vi "FIFO Flush-core.vi"(8 "Error In":errorcluster, 11 "FPGA VI Ref":T1) -> (0 "Error Out":errorcluster, 2 "Ch0 Elements Remaining":u32, 3 "FPGA VI Reference Out":T1)   [LabVIEW 2017]
uses:
  RIG-SPECIFIC FILES/FPGA Refs/FPGA Ref.ctl
  <vilib>/Utility/error.llb/Error Cluster From Error Code.vi
  <vilib>/rvi/errors/niLvFpgaAdjustHostInterfaceError.vi
  <vilib>/rvi/interface/nirviReadWriteControl/nirviReadWriteControl.xnode
  <vilib>/rvi/interface/nirviMethod/nirviMethod.xnode
  <vilib>/rvi/errors/niLvFpgaMergeErrorWithErrorCode.vi
  <vilib>/FPGAPlugInAG/Dynamic/niLvFpga_ReadFifo_Dynamic.vi
  NiFpgaLv.dll
  <vilib>/rvi/interface/Simulation/niFpgaSimulationCallBeginRW.vi
panel:
  out "Loop time array size":i32
  out "Ch1 cleared elements":u32[](array[numeric])
  out "Ch0 Cleared elements":u32[](array[numeric])
  out "Flush Completed":bool
  out "x pixels count":u16[](array[numeric])
  out "y count array":u16[](array[numeric])
  out "x pixels current":u16
  out "y count":u16
  out "Loop Time Array":u32[](array[numeric])
  out "Image time zero":u32
  out "Data Image Time":u64[](array[numeric])
  out "Data Ref Time FIFO":u64[](array[numeric])
  out "Ref time zero":u32
  out "Data Ch1":u32[](array[numeric])
  out "Ch1 Elements Remaining":u32
  out "Data Ch0":u32[](array[numeric])
  in  "Manual force stop":bool
  out "Loop":i32
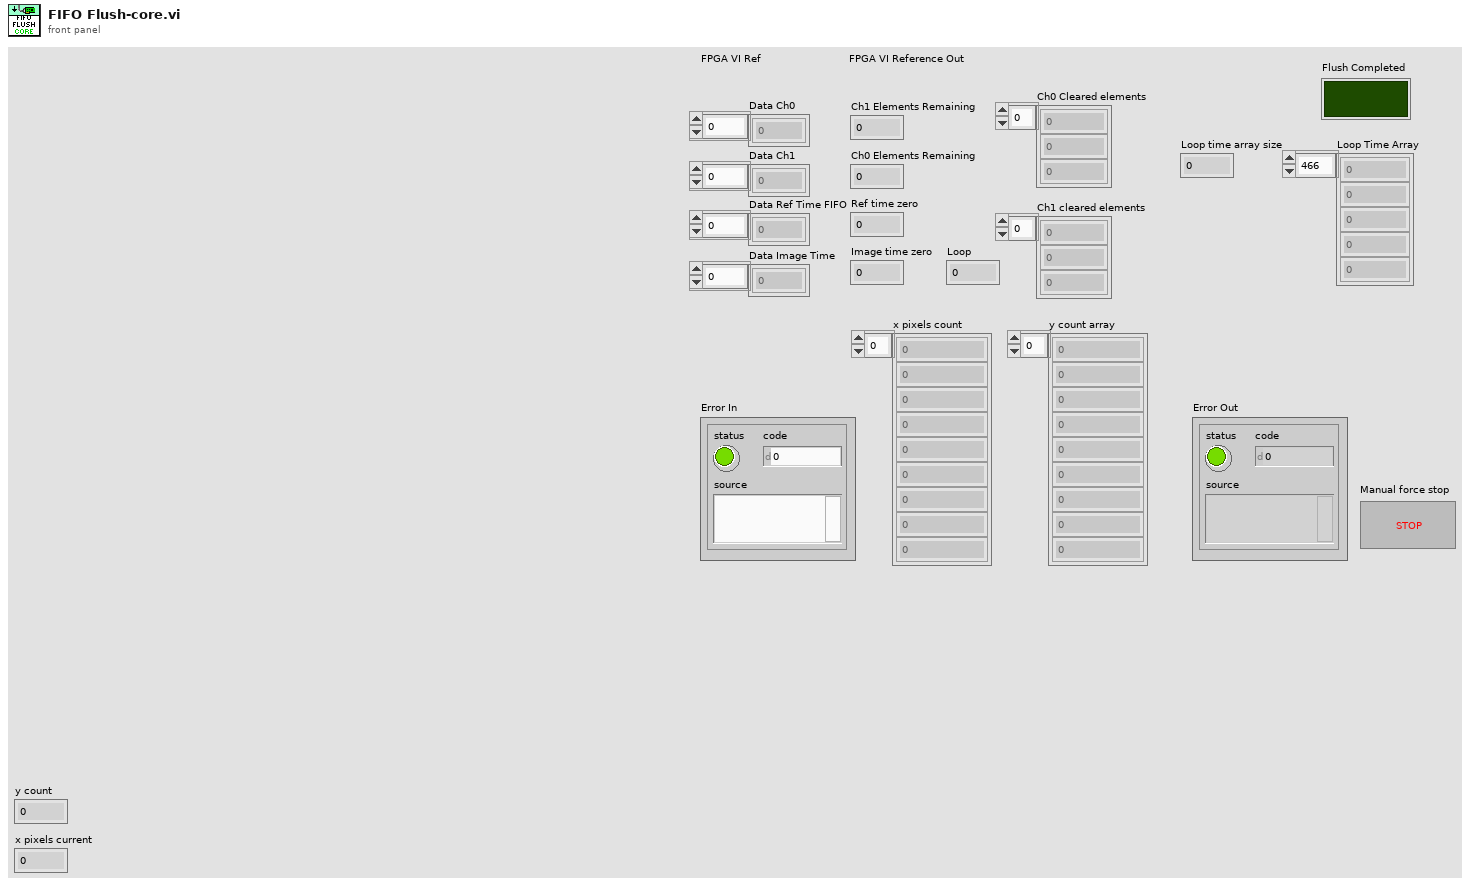
[diagram p1: front panel]
types:
  T1 = typedef "FPGA Ref.ctl" = refnum<k20>
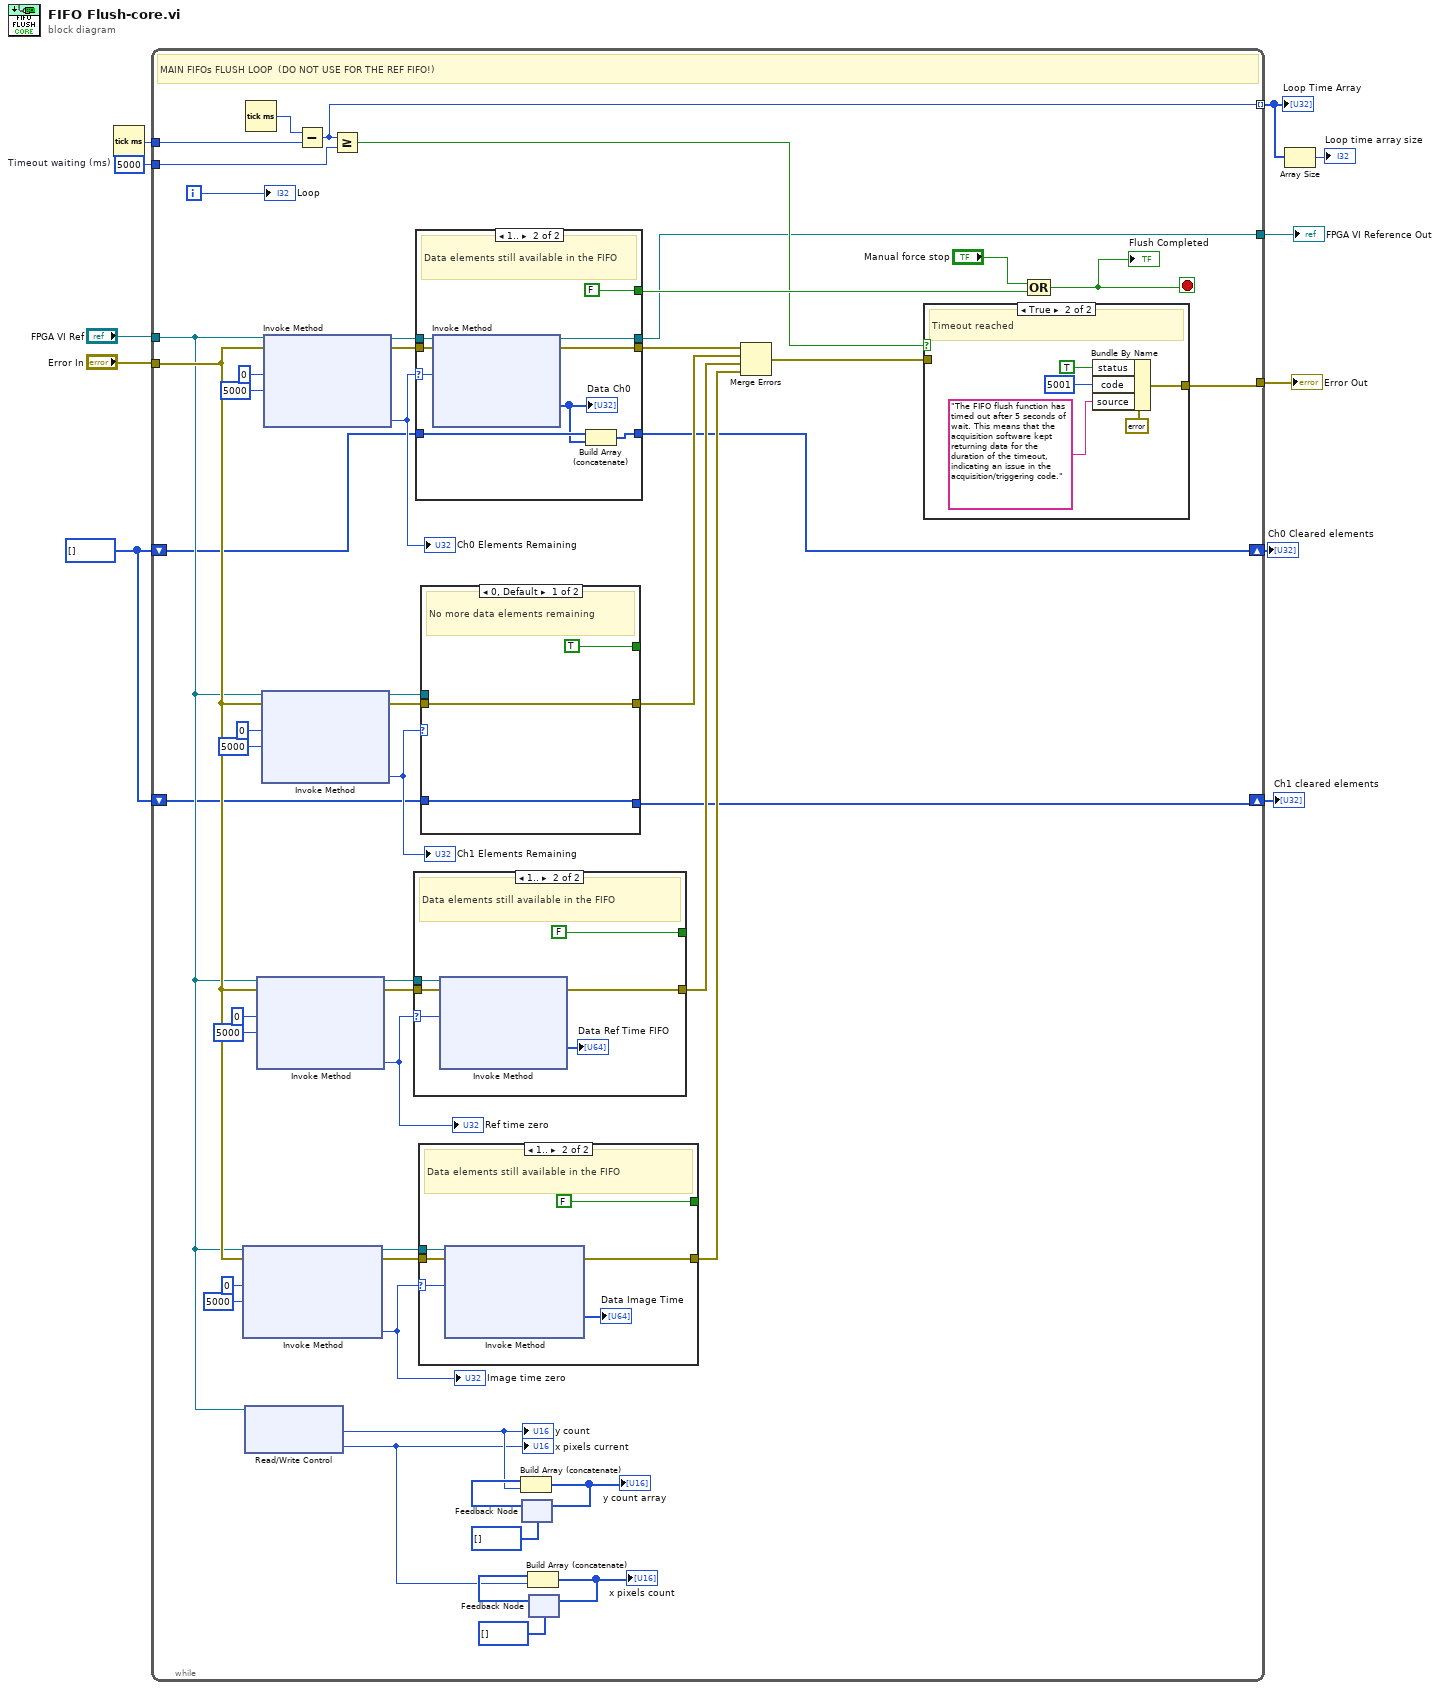
[diagram p0: block diagram]
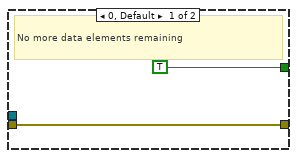
[diagram p2: hidden frame]
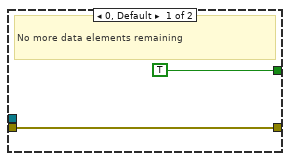
[diagram p3: hidden frame]
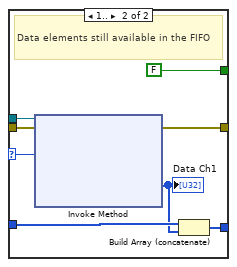
[diagram p4: hidden frame]
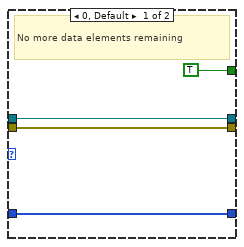
[diagram p6: hidden frame]
diagram:
  w4 = u32[] []
  w7 = u32 5000  # Timeout waiting (ms)
  n1 = Tick Count (ms)() -> (millisecond timer value=w6:u32)
  n2 = while {
    tunnel: "Error In" -> [w27]
    tunnel: [w54] -> w10
    tunnel: w6 -> [w57]
    tunnel: w7 -> [w55]
    tunnel: "FPGA VI Ref" -> [w17]
    tunnel: [w40] -> w8
    tunnel: [w26] -> w2 mode=indexing
    shift-right: [w14] -> w5
    shift-left: w4 -> [w15]
    shift-right: [w12] -> w3
    shift-left: w4 -> [w13]
    i -> [w61]
    stop <- w16 stop-if-true
    # "MAIN FIFOs FLUSH LOOP  (DO NOT USE FOR THE REF FIFO!)"
    n3 = xnode "Invoke Method"("FPGA VI Reference In"=w17, "error in"=w27, "Number of Elements"=u32 0, "Timeout (ms)"=5000) -> ("FPGA VI Reference Out"=w33:T1, "error out"=w34:errorcluster, "Elements Remaining"=w30:u32)  [unwired: 1 out]
    "Image time zero" <- w30
    n4 = xnode "Read/Write Control"("FPGA VI Reference In"=w17) -> ("y count"=w23:u16, "x pixels current"=w18:u16)  [unwired: 1 in, 2 out]
    "y count" <- w23
    "x pixels current" <- w18
    n5 = Tick Count (ms)() -> (millisecond timer value=w58:u32)
    n6 = xnode "Invoke Method"("FPGA VI Reference In"=w17, "error in"=w27, "Number of Elements"=u32 0, "Timeout (ms)"=5000) -> ("FPGA VI Reference Out"=w36:T1, "error out"=w35:errorcluster, "Elements Remaining"=w39:u32)  [unwired: 1 out]
    "Ref time zero" <- w39
    n7 = xnode "Invoke Method"("FPGA VI Reference In"=w17, "error in"=w27, "Number of Elements"=u32 0, "Timeout (ms)"=5000) -> ("FPGA VI Reference Out"=w46:T1, "error out"=w45:errorcluster, "Elements Remaining"=w49:u32)  [unwired: 1 out]
    "Ch1 Elements Remaining" <- w49
    n8 = xnode "Invoke Method"("FPGA VI Reference In"=w17, "error in"=w27, "Number of Elements"=u32 0, "Timeout (ms)"=5000) -> ("FPGA VI Reference Out"=w59:T1, "error out"=w60:errorcluster, "Elements Remaining"=w50:u32)  [unwired: 1 out]
    "Ch0 Elements Remaining" <- w50
    n9 = Subtract(x=w58, y=w57) -> (x-y=w26:u32)
    n10 = Greater Or Equal?(x=w26, y=w55) -> (x >= y?=w41:bool)
    n11 = case shown="1.." w39 {
      selector: w39 -> [_ w74]
      tunnel: w35 -> [w70 w77]
      tunnel: w36 -> [_ w76]
      tunnel: [w70 w75] -> w29
      tunnel: [TRUE FALSE] -> _
      frame 0, Default {
        # "No more data elements remaining"
      }
      frame 1.. {
        # "Data elements still available in the FIFO"
        n12 = xnode "Invoke Method"("FPGA VI Reference In"=w76, "error in"=w77, "Number of Elements"=w74) -> ("error out"=w75:errorcluster, "Data"=→"Data Ref Time FIFO":u64[])  [unwired: 1 in, 2 out]
      }
    }
    n13 = case shown="1.." w50 {
      selector: w50 -> [_ w104]
      tunnel: w60 -> [w97 w107]
      tunnel: w59 -> [w96 w106]
      tunnel: [w97 w105] -> w43
      tunnel: [TRUE FALSE] -> w56
      tunnel: [w96 w102] -> w40
      tunnel: w15 -> [w95 w101]
      tunnel: [w95 w99] -> w14
      frame 0, Default {
        # "No more data elements remaining"
      }
      frame 1.. {
        # "Data elements still available in the FIFO"
        n14 = xnode "Invoke Method"("FPGA VI Reference In"=w106, "error in"=w107, "Number of Elements"=w104) -> ("FPGA VI Reference Out"=w102:T1, "error out"=w105:errorcluster, "Data"=w100:u32[])  [unwired: 1 in, 1 out]
        "Data Ch0" <- w100
        n15 = Build Array (concatenate)(w101, w100) -> (w99:u32[])
      }
    }
    n16 = case shown="1.." w30 {
      selector: w30 -> [_ w66]
      tunnel: w34 -> [w62 w69]
      tunnel: w33 -> [_ w68]
      tunnel: [w62 w67] -> w28
      tunnel: [TRUE FALSE] -> _
      frame 0, Default {
        # "No more data elements remaining"
      }
      frame 1.. {
        # "Data elements still available in the FIFO"
        n17 = xnode "Invoke Method"("FPGA VI Reference In"=w68, "error in"=w69, "Number of Elements"=w66) -> ("error out"=w67:errorcluster, "Data"=→"Data Image Time":u64[])  [unwired: 1 in, 2 out]
      }
    }
    n18 = case shown="0, Default" w49 {
      selector: w49 -> [_ w85]
      tunnel: w45 -> [w79 w88]
      tunnel: w46 -> [_ w87]
      tunnel: [w79 w86] -> w44
      tunnel: [TRUE FALSE] -> _
      tunnel: w13 -> [w78 w83]
      tunnel: [w78 w81] -> w12
      frame 0, Default {
        # "No more data elements remaining"
      }
      frame 1.. {
        # "Data elements still available in the FIFO"
        n19 = xnode "Invoke Method"("FPGA VI Reference In"=w87, "error in"=w88, "Number of Elements"=w85) -> ("error out"=w86:errorcluster, "Data"=w82:u32[])  [unwired: 1 in, 2 out]
        "Data Ch1" <- w82
        n20 = Build Array (concatenate)(w83, w82) -> (w81:u32[])
      }
    }
    n21 = feedback #1(u16[] []) -> (w24:u16[])
    n22 = Build Array (concatenate)(w24, w23) -> (w22:u16[])
    "y count array" <- w22
    n23 = feedback-in #1(w22) -> ()
    n24 = feedback #2(u16[] []) -> (w20:u16[])
    n25 = Build Array (concatenate)(w20, w18) -> (w21:u16[])
    "x pixels count" <- w21
    n26 = feedback-in #2(w21) -> ()
    n27 = Merge Errors(w43, w44, w29, w28) -> (w42:errorcluster)
    n28 = case shown="True" w41 {
      tunnel: w42 -> [w89 _]
      tunnel: [w89 w90] -> w54
      frame False {
      }
      frame True {
        # "Timeout reached"
        n29 = Bundle By Name(cluster=errorcluster {"status"=TRUE, "code"=5001, "source"=""} ("error out"), "status"=TRUE, "code"=5001, "source"="The FIFO flush function has timed out after 5 seconds of wait. This means that the acquisition software kept returning data for the duration of the timeout, indicating an issue in the acquisition/triggering code." ("Error Source")) -> (w90:errorcluster)
      }
    }
    n30 = Compound Arithmetic op=OR("Manual force stop", w56) -> (w16:bool)
    "Flush Completed" <- w16
    "Loop" <- w61
  }
  "Error Out" <- w10
  "FPGA VI Reference Out" <- w8
  "Loop Time Array" <- w2
  "Ch0 Cleared elements" <- w5
  "Ch1 cleared elements" <- w3
  n31 = Array Size(array=w2) -> (size(s)=→"Loop time array size":i32)
